vi "Close RT Sequence.vi"(8 "error in (no error)":errorcluster, 11 "RT Sequence Ref in":refnum<k24>) -> (0 "error out":errorcluster)   [LabVIEW 2016, in "RT Sequence Creator API.lvlib"]
uses:
  RT Sequence Creator API.lvlib
  NationalInstruments.VeriStand.RealTimeSequenceDefinitionApi
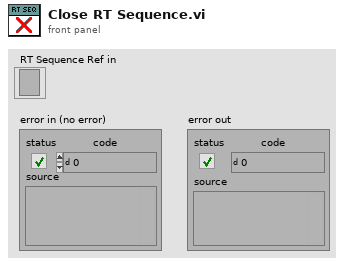
[diagram p1: front panel]
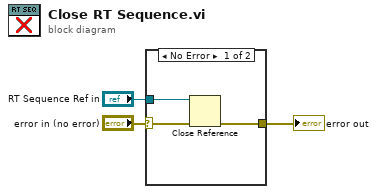
[diagram p0: block diagram]
diagram:
  n1 = case shown="No Error" "error in (no error)" {
    selector: "error in (no error)" -> [w6 w7]
    tunnel: "RT Sequence Ref in" -> [w5 _]
    tunnel: [w4 w7] -> w1
    frame No Error {
      n2 = Close Reference(reference=w5, error in (no error)=w6) -> (error out=w4:errorcluster)
    }
    frame Error {
    }
  }
  "error out" <- w1
